vi "MeasSingleVoltCont.vi"   [LabVIEW 2014]
uses:
  Controls/measVoltState.ctl
  <vilib>/Platform/TimedLoop/XDataNode/timing_clust.ctl
  <vilib>/Platform/TimedLoop/XDataNode/nitl_modes.ctl
  <vilib>/Platform/TimedLoop/XDataNode/wakeup.ctl
  <vilib>/rvi/Emulation/niFpgaGetClockAttributes.vi
  <vilib>/rvi/Emulation/niFpgaSctlEmulationGetInTimedLoop.vi
  <vilib>/rvi/Emulation/niFpgaEmulationReportErrorSimple.vi
  <vilib>/rvi/Emulation/niFpgaCriticalErrorInLSC.vi
  <vilib>/rvi/eio/common/nirviEmuTemplateMethod_errors.vi
  <vilib>/rvi/Emulation/niFpgaEmulationIsFPGAContextNoSignature.vi
  <vilib>/rvi/DataTransferAndStorage/Container/Common/niFpgaContainerGetUniqueNameForEmu.vi
  <vilib>/rvi/eio/common/nirviEmuReportErrorAndStop.vi
  <vilib>/rvi/Emulation/niFpgaProcessEmulError.vi
  measVoltGlobVars.vi
  <vilib>/Platform/TimedLoop/XDataNode/XDataNode.xnode
  <vilib>/eio/EIONode/EIONode.xnode
  <vilib>/rvi/DataTransferAndStorage/Container/XNode/niFpgaContainer.xnode
  <vilib>/rvi/DataTransferAndStorage/Handshake/Emulation/niFpgaHandshakeEmulation.vi
  <vilib>/Platform/TimedLoop/XDataNode/XDNodeRunTimeDep.lvlib
types:
  T1 = typedef "measVoltState.ctl" = enum16{"Idle", "sendMeasRequest", "waitUntilDone", "done"}
  T2 = typedef "XDNodeRunTimeDep.lvlib/timing_clust.ctl" = cluster{"Expected End [f-1]":u64, "Actual End [f-1]":u64, "Finished Late? [f-1]":bool, "Expected End [i-1]":u64, "Actual End [i-1]":u64, "Finished Late? [i-1]":bool, "Expected Start [i]":u64, "Actual Start [i]":u64, "Expected Start [f]":u64, "Actual Start [f]":u64, "Source Name":string, "Structure Name":string, "Period":i64, "Deadline":i64, "Offset":i64, "Start":i64, "Priority":i32, "Timeout":i32, "Mode":T3, "Wakeup Reason":T4, "Error":errorcluster, "Source Type":string, "Secondary Source Type":string, "Global End Time":u64, "Global Start Time":u64, "Frame Duration":u64, "Iteration Duration":u64, "Assigned CPU":i32, "I/O Scan Engine Mode":u32}
  T3 = typedef "XDNodeRunTimeDep.lvlib/nitl_modes.ctl" = enum32{"No Change", "Process missed periods, maintain original phase", "Discard missed periods, maintain original phase", "Process missed periods, ignore original phase", "Discard missed periods, ignore original phase"}
  T4 = typedef "XDNodeRunTimeDep.lvlib/wakeup.ctl" = enum32{"Normal", "Aborted", "Asynchronous wakeup", "Timing source error", "Timed loop error", "Timeout"}
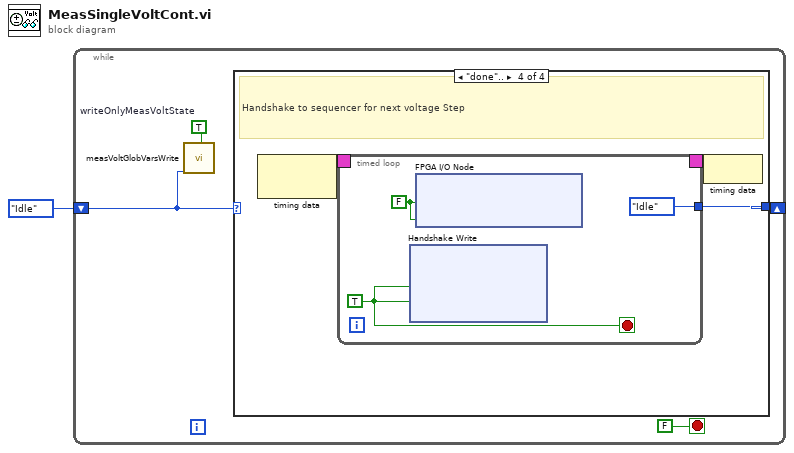
[diagram p0: block diagram]
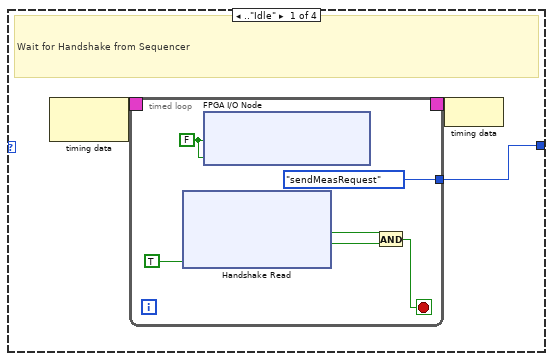
[diagram p2: hidden frame]
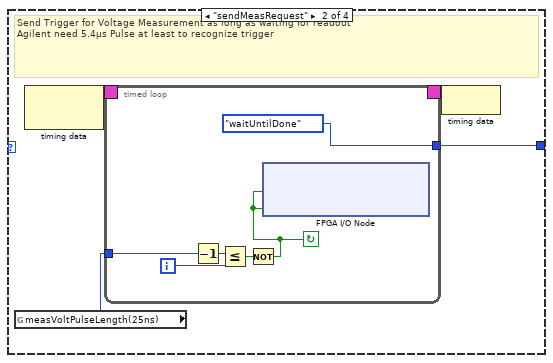
[diagram p3: hidden frame]
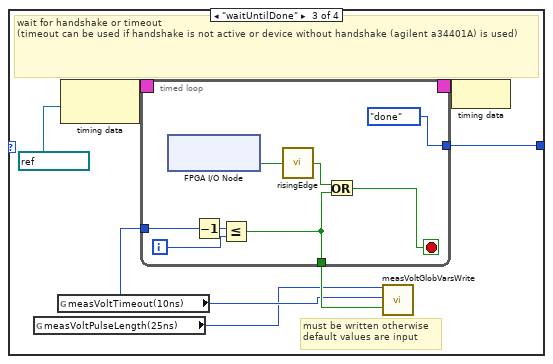
[diagram p4: hidden frame]
diagram:
  n1 = while {
    shift-right: [w4] -> _
    shift-left: measVoltState."Idle" ("measVoltState") -> [w3]
    stop <- FALSE stop-if-true
    w2 = TRUE  # writeOnlyMeasVoltState
    n2 = call "measVoltGlobVarsWrite.vi"("measVoltState"=w3, "writeOnlyMeasVoltState"=w2) -> ()  [unwired: 18 in]
    n3 = case shown="\"done\".." w3 {
      tunnel: [w6 w19 w36 w54] -> w4
      frame .."Idle" {
        # "Wait for Handshake from Sequencer"
        n4 = node-c288() -> (w8:T2)  [unwired: 1 in]
        n5 = timed-loop {
          timing: w8 -> [_]
          timing-out: [_] -> w7
          tunnel: [measVoltState."sendMeasRequest" ("measVoltState")] -> w6
          stop <- w11 stop-if-true
          w9 = FALSE ("PXI_Trig3")
          n6 = xnode ("Handshake Read")("Ready for Output"=TRUE) -> ("Data"=w13:bool, "Output Valid"=w12:bool)  [unwired: 1 in, 1 out]
          n7 = xnode "FPGA I/O Node"("PXI_Trig3"=w9, "measVoltFlagDio8Con1"=w9) -> ()  [unwired: 2 in, 2 out]
          n8 = And(x=w13, y=w12) -> (x .and. y?=w11:bool)
        }
        n9 = node-c288(w7) -> ()
      }
      frame "sendMeasRequest" {
        # "Send Trigger for Voltage Measurement as long as waiting for readout\nAgilent need 5.4µs Pulse at least to recognize trigger"
        n10 = global read "measVoltGlobVars.vi" "measVoltPulseLength(25ns)"() -> (w20:i32)
        n11 = node-c288() -> (w22:T2)  [unwired: 1 in]
        n12 = timed-loop {
          timing: w22 -> [_]
          timing-out: [_] -> w21
          tunnel: w20 -> [w24]
          tunnel: [measVoltState."waitUntilDone" ("measVoltState")] -> w19
          i -> [w28]
          stop <- w25 continue-if-true
          n13 = Decrement(x=w24) -> (x-1=w27:i32)
          n14 = Less Or Equal?(x=w27, y=w28) -> (x <= y?=w26:bool)
          n15 = Not(x=w26) -> (.not. x?=w25:bool)
          n16 = xnode "FPGA I/O Node"("PXI_Trig3"=w25, "measVoltFlagDio8Con1"=w25) -> ()  [unwired: 2 in, 2 out]
        }
        n17 = node-c288(w21) -> ()
      }
      frame "waitUntilDone" {
        # "must be written otherwise\ndefault values are input"
        # "wait for handshake or timeout \n(timeout can be used if handshake is not active or device without handshake (agilent a34401A) is used)"
        n18 = global read "measVoltGlobVars.vi" "measVoltPulseLength(25ns)"() -> (w33:i32)
        n19 = global read "measVoltGlobVars.vi" "measVoltTimeout(10ns)"() -> (w34:i32)
        n20 = node-c288(refnum<k21> "100MHz" ("Source Name")) -> (w39:T2)
        n21 = timed-loop {
          timing: w39 -> [_]
          timing-out: [_] -> w38
          tunnel: w34 -> [w46]
          tunnel: [w41] -> w37
          tunnel: [measVoltState."done" ("measVoltState")] -> w36
          i -> [w45]
          stop <- w44 stop-if-true
          n22 = xnode "FPGA I/O Node"() -> ("PXI_Trig4"=w43:bool)  [unwired: 1 in, 1 out]
          n23 = Decrement(x=w46) -> (x-1=w47:i32)
          n24 = Less Or Equal?(x=w47, y=w45) -> (x <= y?=w41:bool)
          n25 = call "risingEdge.vi"("In"=w43) -> ("out"=w42:bool)
          n26 = Or(x=w42, y=w41) -> (x .or. y?=w44:bool)
        }
        n27 = call "measVoltGlobVarsWrite.vi"("measVoltPulseLength(25ns)"=w33, "measVoltTimeout(10ns)"=w34, "timedOutWhileHandshake"=w37) -> ()  [unwired: 17 in]
        n28 = node-c288(w38) -> ()
      }
      frame "done".. {
        # "Handshake to sequencer for next voltage Step"
        n29 = node-c288() -> (w56:T2)  [unwired: 1 in]
        n30 = timed-loop {
          timing: w56 -> [_]
          timing-out: [_] -> w55
          tunnel: [measVoltState."Idle" ("measVoltState")] -> w54
          stop <- w59 stop-if-true
          w57 = FALSE ("PXI_Trig3")
          w59 = TRUE ("Ready for Output")
          n31 = xnode ("Handshake Write")("Data"=w59, "Input Valid"=w59) -> ()  [unwired: 1 in, 2 out]
          n32 = xnode "FPGA I/O Node"("PXI_Trig3"=w57, "measVoltFlagDio8Con1"=w57) -> ()  [unwired: 2 in, 2 out]
        }
        n33 = node-c288(w55) -> ()
      }
    }
  }
